vi "Read channels.vi"(8 "error in (no error)":errorcluster, 11 "Conditional Jump Step Config in":refnum<class "Conditional Jump Step Config.lvclass">) -> (0 "error out":errorcluster, 2 "Channels":refnum<class "TBM channel.lvclass">[](array[class]), 3 "Conditional Jump Step Config out":refnum<class "Conditional Jump Step Config.lvclass">)   [LabVIEW 2015, in "Conditional Jump Step Config.lvclass"]
uses:
  Conditional Jump Step Config.lvclass
  <vilib>/NI/Tag Bus Module Framework/channel/TBM channel.lvclass
  Conditional Jump Step Config.lvclass/Conditional Jump Step Config.ctl
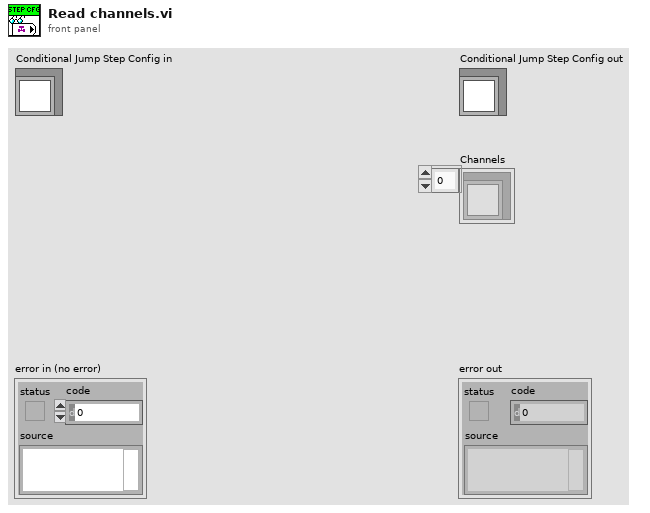
[diagram p1: front panel]
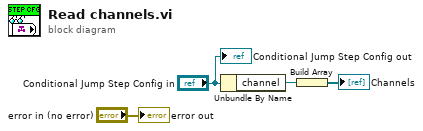
[diagram p0: block diagram]
diagram:
  n1 = Unbundle By Name("Conditional Jump Step Config in") -> ("channel"=w1:refnum<class "TBM channel.lvclass">)
  n2 = Build Array(w1) -> (→"Channels":refnum<class "TBM channel.lvclass">[])
  "error out" <- "error in (no error)"
  "Conditional Jump Step Config out" <- "Conditional Jump Step Config in"
